vi "format floats for database.vi"(4 "Number":dbl) -> (1 "Insertion String":string)   [LabVIEW 2014, in "hse-db.lvlib" / "ADO-DB-Driver.lvlib"]
uses:
  ADO-DB-Driver.lvlib
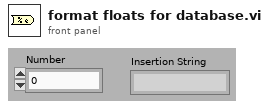
[diagram p1: front panel]
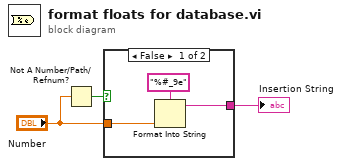
[diagram p0: block diagram]
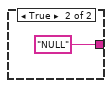
[diagram p2: hidden frame]
diagram:
  n1 = Not A Number/Path/Refnum?(number/path/refnum="Number") -> (NaN/Path/Refnum?=w3:bool)
  n2 = case shown="False" w3 {
    tunnel: "Number" -> [w5 _]
    tunnel: [w4 "NULL"] -> w2
    frame False {
      n3 = Format Into String(format string="%#_9e", w5) -> (resulting string=w4:string)  [unwired: 2 in, 1 out]
    }
    frame True {
    }
  }
  "Insertion String" <- w2
